vi "TPNT_DBSCore.vi"(0 "Object Refnum In":T6, 1 "Name":string, 2 "Object Data In":T1={"device"="", "devupdate"=0.0, "next_update"=0, "devinterface"="", "TPs"=[], "Alarms"=TRUE, "monitor"=TRUE, "log sep"=""} {"TPs"."Log"."updaterate" format="%.2f"; "TPs"."Samples"."Values" format="%.2f"; "TPs"."Samples"."samples" min=1 step=1; "TPs"."Limits"."Nominal" format="%.2f"; "TPs"."Limits"."Upper" format="%.2f"; "TPs"."Limits"."Lower" format="%.2f"; "TPs"."update_rate" format="%.2f"; "devupdate" format="%.2f"}, 5 "error in (no error)":errorcluster, 6 "Function (Get Data)":T7=enum."Get Data") -> (11 "Valid Object":bool, 12 "Objects":T6[](array[typedef]), 13 "Created New":bool, 14 "Object Refnum out":T6, 15 "Name Out":string, 16 "Object Data Out":T1={"device"="", "devupdate"=0.0, "next_update"=0, "devinterface"="", "TPs"=[], "Alarms"=TRUE, "monitor"=TRUE, "log sep"=""} {"TPs"."Log"."updaterate" format="%.2f"; "TPs"."Samples"."Values" format="%.2f"; "TPs"."Samples"."samples" min=1 step=1; "TPs"."Limits"."Nominal" format="%.2f"; "TPs"."Limits"."Upper" format="%.2f"; "TPs"."Limits"."Lower" format="%.2f"; "TPs"."update_rate" format="%.2f"; "devupdate" format="%.2f"}, 19 "error out":errorcluster)   [LabVIEW 2016]
doc: "This VI is the object core. It assigns a RefNum for each object as it is created using the Register function. Object data is accessed using the appropriate RefNum.\nCopyright 2001 VI Engineering, Inc."
uses:
  TPNT_Refnum.ctl
  TPNT_CoreFunction.ctl
  TPNT_DeviceTPs.ctl
  TPNT_TP.ctl
  TPNT_Limits.ctl
  TPNT_Samples.ctl
  TPNT_Log.ctl
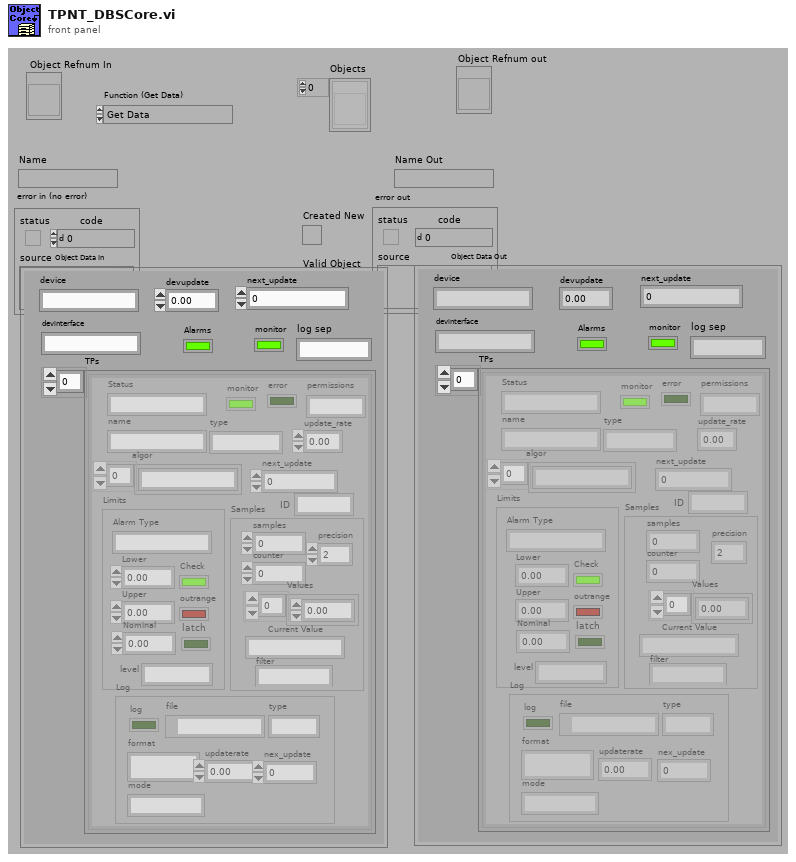
[diagram p1: front panel]
types:
  T1 = typedef "TPNT_DeviceTPs.ctl" = cluster{"device":string, "devupdate":dbl, "next_update":u32, "devinterface":string, "TPs":T2[], "Alarms":bool, "monitor":bool, "log sep":string}
  T2 = typedef "TPNT_TP.ctl" = cluster{"name":string, "type":string, "algor":string[], "update_rate":sgl, "Limits":T3, "Samples":T4, "next_update":u32, "Status":string, "monitor":bool, "error":bool, "Log":T5, "permissions":string, "ID":string}
  T3 = typedef "TPNT_Limits.ctl" = cluster{"Alarm Type":string, "Lower ":dbl, "Upper":dbl, "Nominal":dbl, "outrange":bool, "Check":bool, "latch":bool, "level":string}
  T4 = typedef "TPNT_Samples.ctl" = cluster{"samples":i32, "counter":i32, "Values":dbl[], "Current Value":string, "filter":string, "precision":u8}
  T5 = typedef "TPNT_Log.ctl" = cluster{"log":bool, "file":path, "type":string, "format":string, "updaterate":dbl, "nex_update":u32, "mode":string}
  T6 = typedef "TPNT_Refnum.ctl" = refnum<vi>
  T7 = typedef "TPNT_CoreFunction.ctl" = enum16{"Reset", "Register", "Get Data", "Set Data", "Unregister", "Test", "Get Objects"}
  T8 = typedef "Semaphore RefNum" = refnum<k1>
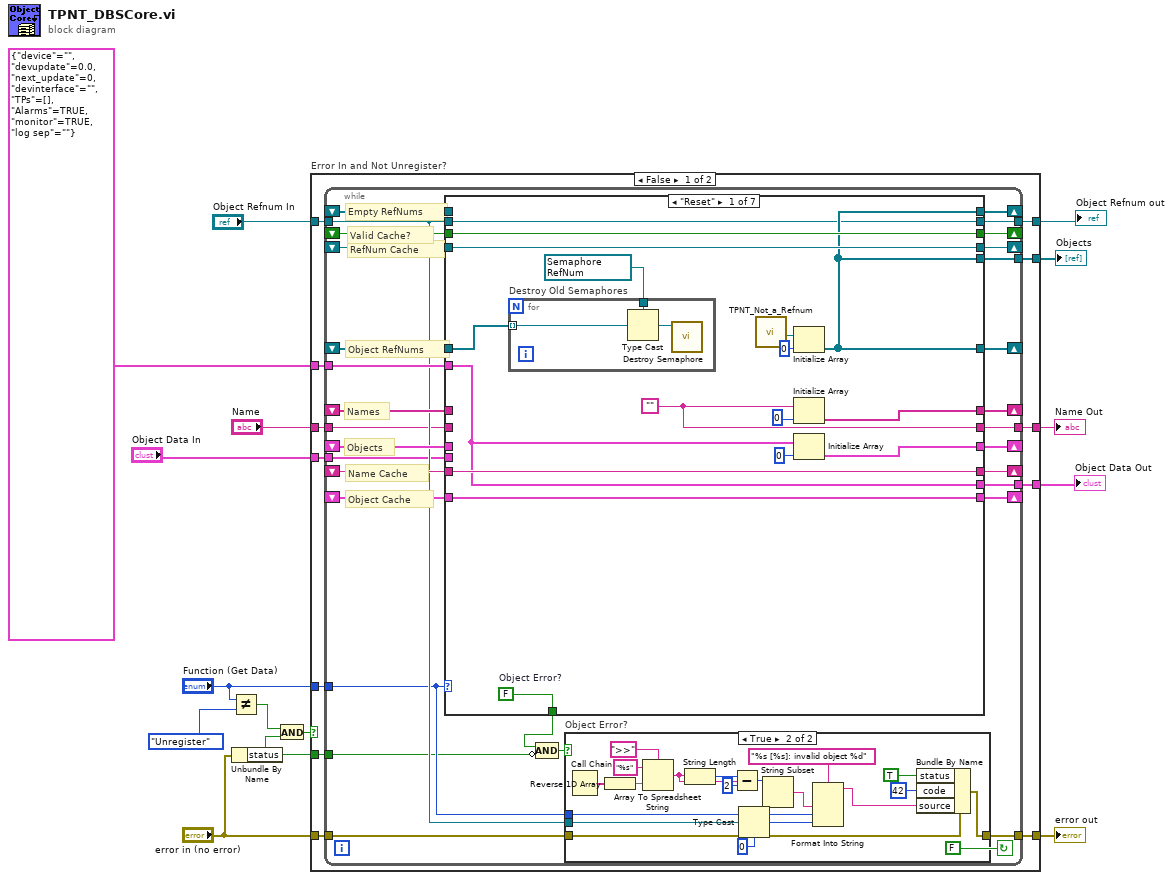
[diagram p0: block diagram]
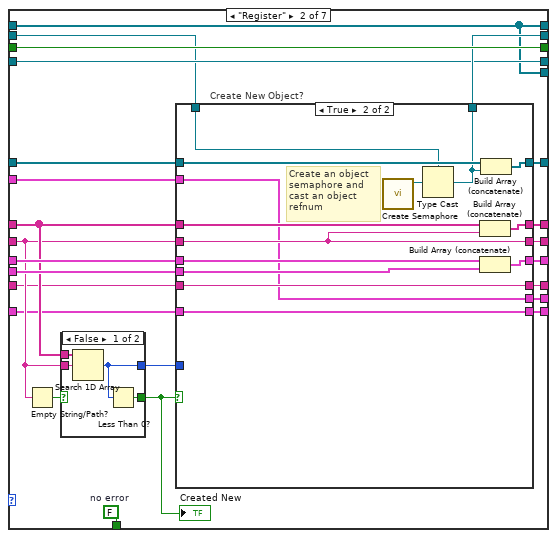
[diagram p3: hidden frame]
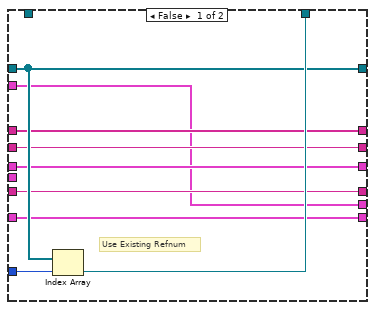
[diagram p4: hidden frame]
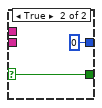
[diagram p5: hidden frame]
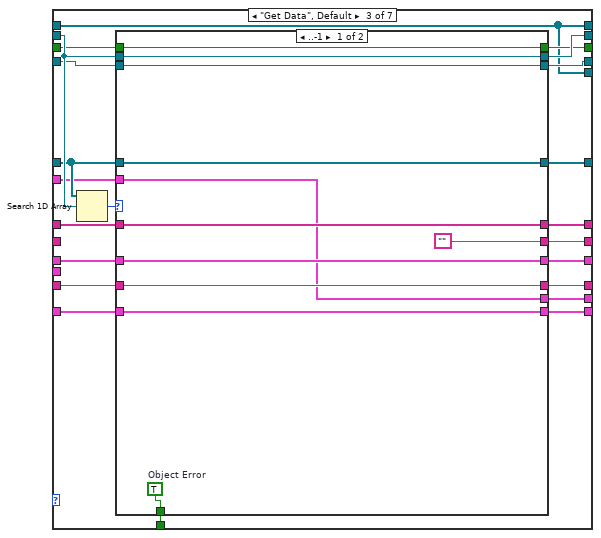
[diagram p6: hidden frame]
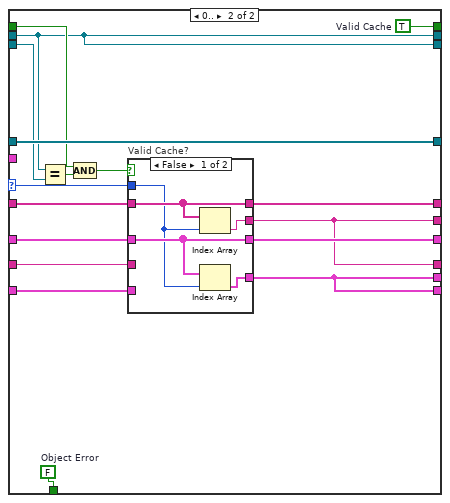
[diagram p7: hidden frame]
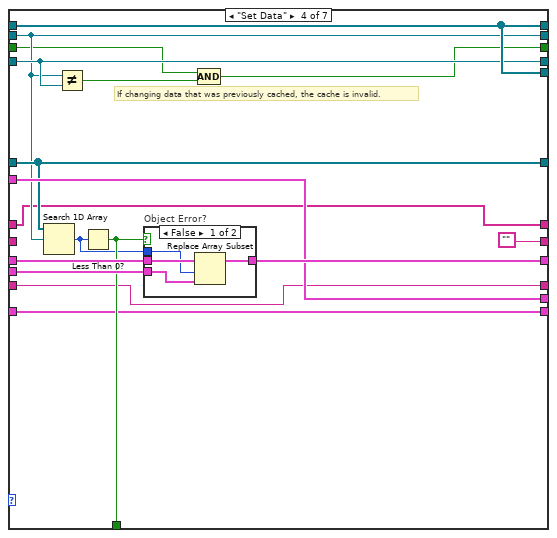
[diagram p9: hidden frame]
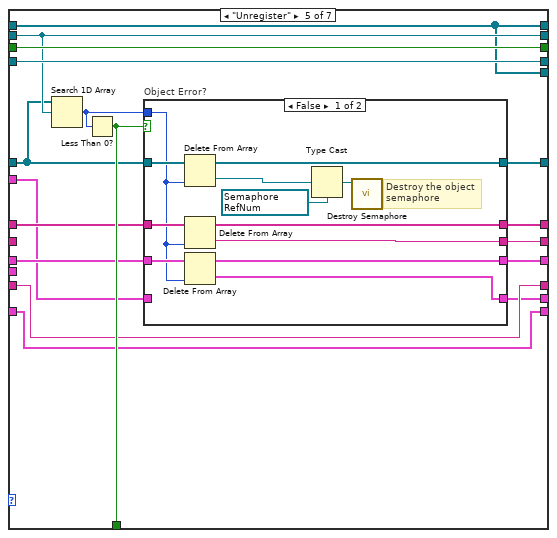
[diagram p11: hidden frame]
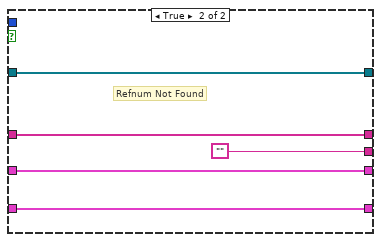
[diagram p12: hidden frame]
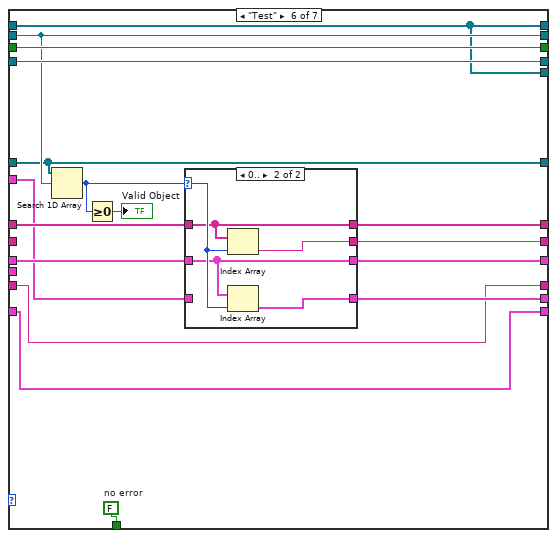
[diagram p13: hidden frame]
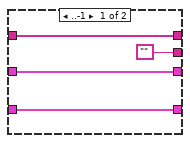
[diagram p14: hidden frame]
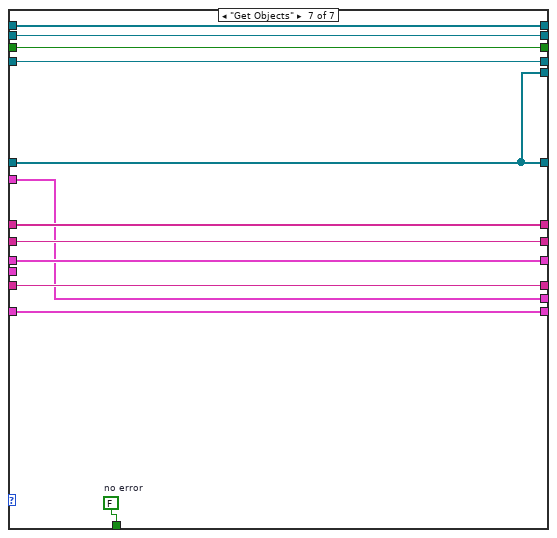
[diagram p15: hidden frame]
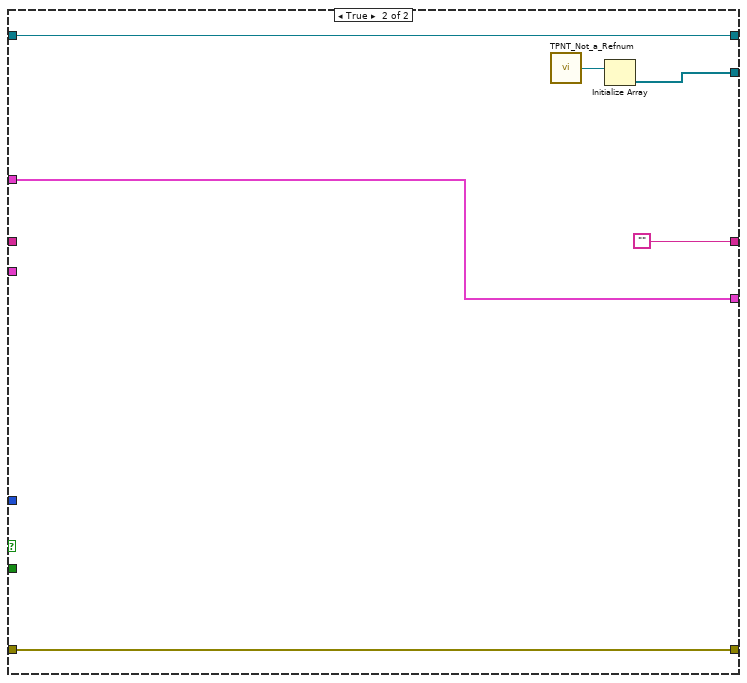
[diagram p16: hidden frame]
diagram:
  n1 = Not Equal?(x="Function (Get Data)", y=TPNT_CoreFunction."Unregister" ("Function (Get Data)")) -> (x != y?=w9:bool)
  n2 = Unbundle By Name("error in (no error)") -> ("status"=w10:bool)
  n3 = And(x=w9, y=w10) -> (x .and. y?=w8:bool)
  n4 = case "Error In and Not Unregister?" shown="False" w8 {
    tunnel: "Object Refnum In" -> [w27 w309]
    tunnel: T1 {"device"="", "devupdate"=0.0, "next_update"=0, "devinterface"="", "TPs"=[], "Alarms"=TRUE, "monitor"=TRUE, "log sep"=""} ("Object Data In") -> [w26 w305]
    tunnel: "error in (no error)" -> [w25 w310]
    tunnel: [w24 w310] -> w15
    tunnel: "Object Data In" -> [w23 _]
    tunnel: [w22 w309] -> w6
    tunnel: "Name" -> [w21 _]
    tunnel: [w20 ""] -> w13
    tunnel: [w19 w305] -> w4
    tunnel: [w18 w307] -> w3
    tunnel: "Function (Get Data)" -> [w17 _]
    tunnel: w10 -> [w16 _]
    frame False {
      n5 = while {
        tunnel: w16 -> [w31]
        shift-left: _ -> [w32]
        shift-right: [w33] -> _
        tunnel: [w34] -> w18
        tunnel: [w35] -> w19
        tunnel: [w36] -> w20
        tunnel: w21 -> [w37]
        tunnel: [w38] -> w22
        tunnel: w23 -> [w39]
        tunnel: [w40] -> w24
        tunnel: w25 -> [w43]
        shift-left: _ -> [w46]
        shift-right: [w45] -> _
        shift-left: _ -> [w48]
        shift-right: [w47] -> _
        shift-left: _ -> [w50]
        shift-right: [w49] -> _
        tunnel: w26 -> [w44]
        tunnel: w27 -> [w42]
        shift-left: _ -> [w52]
        shift-right: [w51] -> _
        shift-left: _ -> [w54]
        shift-right: [w53] -> _
        shift-left: _ -> [w56]
        shift-right: [w55] -> _
        shift-left: _ -> [w58]
        shift-right: [w57] -> _
        tunnel: w17 -> [w41]
        stop <- FALSE continue-if-true
        # "Empty RefNums"
        # "Object Cache"
        # "Name Cache"
        # "Names"
        # "Objects"
        # "Object RefNums"
        # "RefNum Cache"
        # "Valid Cache?"
        n6 = case shown="\"Reset\"" w41 {
          tunnel: w42 -> [w83 w113 w172 w216 w247 w281 w302]
          tunnel: w58 -> [w95 w122 w171 w213 w248 w282 w303]
          tunnel: [w95 w122 w165 w215 w248 w282 w303] -> w57
          tunnel: w56 -> [w94 w115 w170 w217 w249 w283 w304]
          tunnel: [w94 w115 w164 w217 w249 w283 w304] -> w55
          tunnel: w54 -> [w79 w114 w169 w219 w245 w280 w293]
          tunnel: [w84 w121 w163 w219 w242 w280 w293] -> w53
          tunnel: w52 -> [_ w120 w168 w226 w243 w276 w296]
          tunnel: [w90 w119 w162 w225 w239 w272 w296] -> w51
          tunnel: w50 -> [_ w112 w167 w214 w244 w277 w298]
          tunnel: [w85 w116 w161 w214 w240 w273 w298] -> w49
          tunnel: w48 -> [w93 w108 w160 w221 w238 w269 w299]
          tunnel: [w93 w107 w156 w221 w238 w269 w299] -> w47
          tunnel: w46 -> [w92 w106 w159 w220 w237 w270 w300]
          tunnel: [w92 w105 w155 w220 w237 w270 w300] -> w45
          tunnel: w44 -> [w81 w102 w153 w223 w233 w271 w295]
          tunnel: [w87 w100 w154 w224 w246 w279 w301] -> w29
          tunnel: w39 -> [_ w118 _ w227 _ _ _]
          tunnel: [w83 w117 w166 w216 w247 w281 w302] -> w38
          tunnel: w37 -> [_ w111 _ _ _ _ w297]
          tunnel: [w82 w104 w158 "" w235 w275 w297] -> w36
          tunnel: [w81 w103 w157 w223 w234 w274 w295] -> w35
          tunnel: [w84 w101 w152 w218 w236 w268 w293] -> w34
          tunnel: [w84 w101 w152 w218 w236 w268 w294] -> w33
          tunnel: w32 -> [_ w101 w152 w218 w236 w268 w294]
          frame "Reset" {
            w80 = T8 refnum items=["semaphore"] ("semaphore")
            w87 = FALSE  # Object Error?
            w82 = ""
            n7 = for "Destroy Old Semaphores" {
              tunnel: w79 -> [w97] mode=indexing
              tunnel: w80 -> [w98]
              n8 = Type Cast(type=w98, x=w97) -> (*(type *) &x=w96:T8)
              n9 = call <vilib>:"Destroy Semaphore.vi"("semaphore"=w96) -> ()  [unwired: 1 in, 6 out]
            }
            n10 = call "TPNT_Not_a_Refnum.vi"() -> ("Not_an_element_Refnum"=w88:T6)
            n11 = Initialize Array(w88, 0 ("Dimension Size")) -> (w84:T6[])
            n12 = Initialize Array(w82, 0 ("Dimension Size")) -> (w85:string[])
            n13 = Initialize Array(w81, 0 ("Dimension Size")) -> (w90:T1[])
          }
          frame "Register" {
            w100 = FALSE  # no error
            n14 = Empty String/Path?(string/path=w111) -> (empty?=w110:bool)
            n15 = case shown="False" w110 {
              selector: w110 -> [_ w151]
              tunnel: w112 -> [w149 _]
              tunnel: w111 -> [w148 _]
              tunnel: [w147 0 ("index of element")] -> w109
              tunnel: [w146 w151] -> w99
              frame False {
                n16 = Search 1D Array(1D array=w149, element=w148) -> (index of element=w147:i32)  [unwired: 1 out]
                n17 = Less Than 0?(x=w147) -> (x < 0?=w146:bool)
              }
              frame True {
              }
            }
            "Created New" <- w99
            n18 = case "Create New Object?" shown="True" w99 {
              tunnel: [w130 w145] -> w121
              tunnel: w120 -> [w127 w144]
              tunnel: [w127 w143] -> w119
              tunnel: w118 -> [_ w142]
              tunnel: [w131 w132] -> w117
              tunnel: [w129 w141] -> w116
              tunnel: w114 -> [w130 w140]
              tunnel: w113 -> [_ w133]
              tunnel: w112 -> [w129 w139]
              tunnel: w111 -> [w128 w136]
              tunnel: w109 -> [w123 _]
              tunnel: w108 -> [w126 w138]
              tunnel: [w126 w138] -> w107
              tunnel: w106 -> [w125 w137]
              tunnel: [w125 w137] -> w105
              tunnel: [w128 w136] -> w104
              tunnel: [w124 w135] -> w103
              tunnel: w102 -> [w124 w135]
              frame False {
                # "Use Existing Refnum"
                n19 = Index Array(array=w130, index=w123) -> (element=w131:T6)
              }
              frame True {
                # "Create an object semaphore and cast an object refnum"
                n20 = call <vilib>:"Create Semaphore.vi"() -> ("semaphore"=w134:T8)  [unwired: 2 in, 5 out]
                n21 = Type Cast(type=w133, x=w134) -> (*(type *) &x=w132:T6)
                n22 = Build Array (concatenate)(w139, w136) -> (w141:string[])
                n23 = Build Array (concatenate)(w144, w142) -> (w143:T1[])
                n24 = Build Array (concatenate)(w140, w132) -> (w145:T6[])
              }
            }
          }
          frame "Get Data", Default {
            n25 = Search 1D Array(1D array=w169, element=w172) -> (index of element=w173:i32)  [unwired: 1 out]
            n26 = case shown="..-1" w173 {
              selector: w173 -> [_ w185]
              tunnel: w172 -> [w180 w190]
              tunnel: w171 -> [w179 w191]
              tunnel: w170 -> [w178 w199]
              tunnel: w169 -> [w177 w201]
              tunnel: w168 -> [w183 w195]
              tunnel: w167 -> [w184 w194]
              tunnel: [w180 w190] -> w166
              tunnel: [w179 w189] -> w165
              tunnel: [w178 w190] -> w164
              tunnel: [w177 w201] -> w163
              tunnel: [w183 w193] -> w162
              tunnel: [w184 w192] -> w161
              tunnel: w160 -> [w181 w197]
              tunnel: w159 -> [w182 w196]
              tunnel: ["" w188] -> w158
              tunnel: [w175 w187] -> w157
              tunnel: [w181 w188] -> w156
              tunnel: [w182 w187] -> w155
              tunnel: [w176 w186] -> w154
              tunnel: w153 -> [w175 _]
              frame ..-1 {
                w176 = TRUE  # Object Error
              }
              frame 0.. {
                w186 = FALSE  # Object Error
                w189 = TRUE  # Valid Cache
                n27 = Equal?(x=w190, y=w199) -> (x = y?=w200:bool)
                n28 = Compound Arithmetic op=AND(w191, w200) -> (w198:bool)
                n29 = case "Valid Cache?" shown="False" w198 {
                  tunnel: w197 -> [_ w210]
                  tunnel: w196 -> [_ w209]
                  tunnel: w195 -> [w204 w208]
                  tunnel: w194 -> [w203 w207]
                  tunnel: [w206 w210] -> w188
                  tunnel: [w205 w209] -> w187
                  tunnel: w185 -> [w202 _]
                  tunnel: [w204 w208] -> w193
                  tunnel: [w203 w207] -> w192
                  frame False {
                    n30 = Index Array(array=w203, index=w202) -> (element=w206:string)
                    n31 = Index Array(array=w204, index=w202) -> (element=w205:T1)
                  }
                  frame True {
                  }
                }
              }
            }
          }
          frame "Set Data" {
            # "If changing data that was previously cached, the cache is invalid."
            n32 = Search 1D Array(1D array=w219, element=w216) -> (index of element=w211:i32)  [unwired: 1 out]
            n33 = Not Equal?(x=w216, y=w217) -> (x != y?=w212:bool)
            n34 = Less Than 0?(x=w211) -> (x < 0?=w224:bool)
            n35 = case "Object Error?" shown="False" w224 {
              tunnel: w227 -> [w230 _]
              tunnel: w226 -> [w231 w232]
              tunnel: [w229 w232] -> w225
              tunnel: w211 -> [w228 _]
              frame False {
                n36 = Replace Array Subset(array=w231, new element=w230, index=w228) -> (w229:T1[])
              }
              frame True {
              }
            }
            n37 = Compound Arithmetic op=AND(w213, w212) -> (w215:bool)
          }
          frame "Unregister" {
            n38 = Search 1D Array(1D array=w245, element=w247) -> (index of element=w241:i32)  [unwired: 1 out]
            n39 = Less Than 0?(x=w241) -> (x < 0?=w246:bool)
            n40 = case "Object Error?" shown="False" w246 {
              tunnel: w245 -> [w261 w264]
              tunnel: w244 -> [w259 w266]
              tunnel: w243 -> [w257 w265]
              tunnel: [w260 w264] -> w242
              tunnel: w241 -> [w253 _]
              tunnel: [w258 w266] -> w240
              tunnel: [w256 w265] -> w239
              tunnel: [w255 ""] -> w235
              tunnel: [w254 w262] -> w234
              tunnel: w233 -> [_ w262]
              frame False {
                w252 = T8 refnum items=["semaphore"] ("semaphore")
                # "Destroy the object semaphore"
                n41 = Delete From Array(array=w261, index=w253) -> (deleted portion=w251:T6, array with subset deleted=w260:T6[])  [unwired: 1 in]
                n42 = Delete From Array(array=w259, index=w253) -> (deleted portion=w255:string, array with subset deleted=w258:string[])  [unwired: 1 in]
                n43 = Delete From Array(array=w257, index=w253) -> (deleted portion=w254:T1, array with subset deleted=w256:T1[])  [unwired: 1 in]
                n44 = Type Cast(type=w252, x=w251) -> (*(type *) &x=w250:T8)
                n45 = call <vilib>:"Destroy Semaphore.vi"("semaphore"=w250) -> ()  [unwired: 1 in, 6 out]
              }
              frame True {
                # "Refnum Not Found"
              }
            }
          }
          frame "Test" {
            w279 = FALSE  # no error
            n46 = Search 1D Array(1D array=w280, element=w281) -> (index of element=w267:i32)  [unwired: 1 out]
            n47 = Greater Or Equal To 0?(x=w267) -> (x >= 0?=→"Valid Object":bool)
            n48 = case shown="0.." w267 {
              selector: w267 -> [_ w292]
              tunnel: w277 -> [w287 w289]
              tunnel: w276 -> [w286 w288]
              tunnel: ["" w291] -> w275
              tunnel: [w284 w290] -> w274
              tunnel: [w287 w289] -> w273
              tunnel: [w286 w288] -> w272
              tunnel: w271 -> [w284 _]
              frame ..-1 {
              }
              frame 0.. {
                n49 = Index Array(array=w289, index=w292) -> (element=w291:string)
                n50 = Index Array(array=w288, index=w292) -> (element=w290:T1)
              }
            }
          }
          frame "Get Objects" {
            w301 = FALSE  # no error
          }
        }
        n51 = Compound Arithmetic op=AND(w29, invert w31) -> (w30:bool)
        n52 = case "Object Error?" shown="True" w30 {
          tunnel: w41 -> [_ w76]
          tunnel: w42 -> [_ w77]
          tunnel: w43 -> [w59 w72]
          tunnel: [w59 w73] -> w40
          frame False {
          }
          frame True {
            n53 = Call Chain() -> (call chain=w71:string[])
            n54 = Reverse 1D Array(array=w71) -> (reversed array=w69:string[])
            n55 = Array To Spreadsheet String(delimiter (Tab)=">>", array=w69, 3:"%s" ("format string")) -> (spreadsheet string=w64:string)
            n56 = String Length(string=w64) -> (length=w67:i32)
            n57 = Subtract(x=w67, y=2) -> (x-y=w65:i32)
            n58 = Type Cast(type=u32 0 ("object"), x=w77) -> (*(type *) &x=w75:u32)
            n59 = String Subset(string=w64, length (rest)=w65) -> (substring=w63:string)  [unwired: 1 out]
            n60 = Format Into String(format string="%s [%s]: invalid object %d", w63, w76, w75) -> (resulting string=w62:string)  [unwired: 2 in, 1 out]
            n61 = Bundle By Name(cluster=w72, "status"=TRUE ("Bundle Element"), "code"=42 ("Bundle Element"), "source"=w62) -> (w73:errorcluster)
          }
        }
      }
    }
    frame True {
      n62 = call "TPNT_Not_a_Refnum.vi"() -> ("Not_an_element_Refnum"=w308:T6)
      n63 = Initialize Array(w308) -> (w307:T6[])  [unwired: 1 out]
    }
  }
  "Objects" <- w3
  "error out" <- w15
  "Name Out" <- w13
  "Object Refnum out" <- w6
  "Object Data Out" <- w4
